vi "Find Names of PNP Devices.vi"(4 "Error In":errorcluster, 7 "Identifiers (regular expressions. Use blank to ignore)":T3={"Service"="FTSER2K", "Manufacturer"="FTDI", "Device"="FTDIBUS", "Vendor ID"="VID_0403", "Product ID"="PID_6001", "S/N"="FTXOVPUUA", "Instance"="0000"}) -> (0 "Error Out":errorcluster, 1 "Matching Items":T1(array[cluster]), 3 "Names":T2(array[cluster]))   [LabVIEW 2016]
doc: "Returns names, captions, & descriptions of PNP devices whose properties match the fields in the 'Identifiers' cluster\nFields are regular expressions (use .* to match any)."
uses:
  System.Management
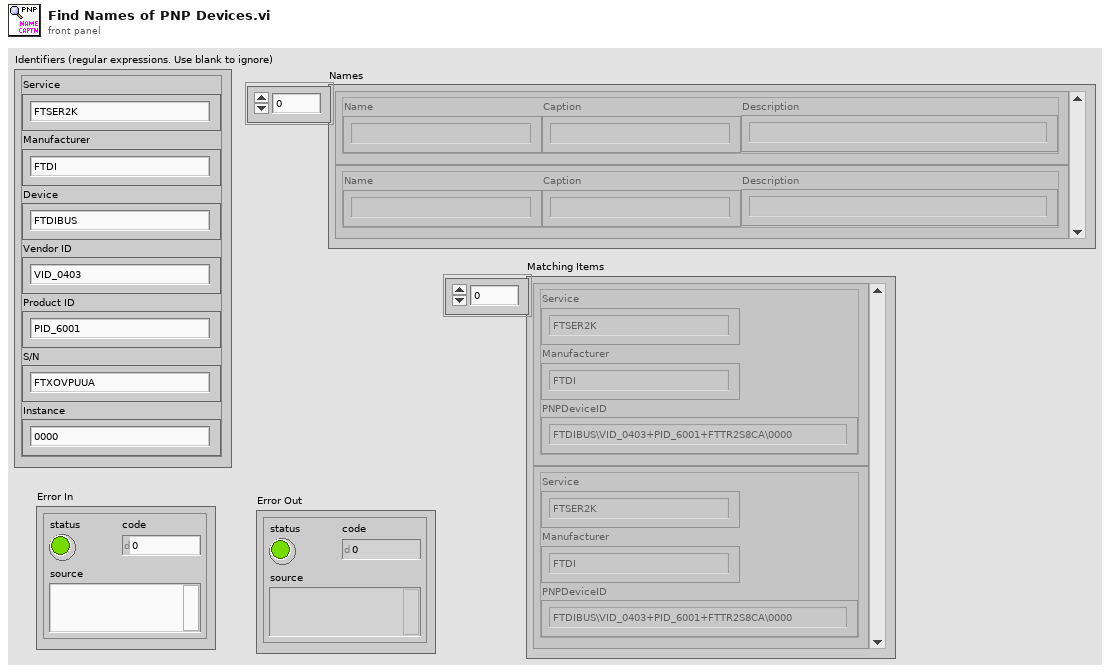
[diagram p1: front panel]
types:
  T1 = cluster{"Service":string, "Manufacturer":string, "PNPDeviceID":string}[]
  T2 = cluster{"Name":string, "Caption":string, "Description":string}[]
  T3 = cluster{"Service":string, "Manufacturer":string, "Device":string, "Vendor ID":string, "Product ID":string, "S/N":string, "Instance":string}
  T4 = cluster{"Property Values[0]":string, "Property Values[1]":string, "Property Values[2]":string}
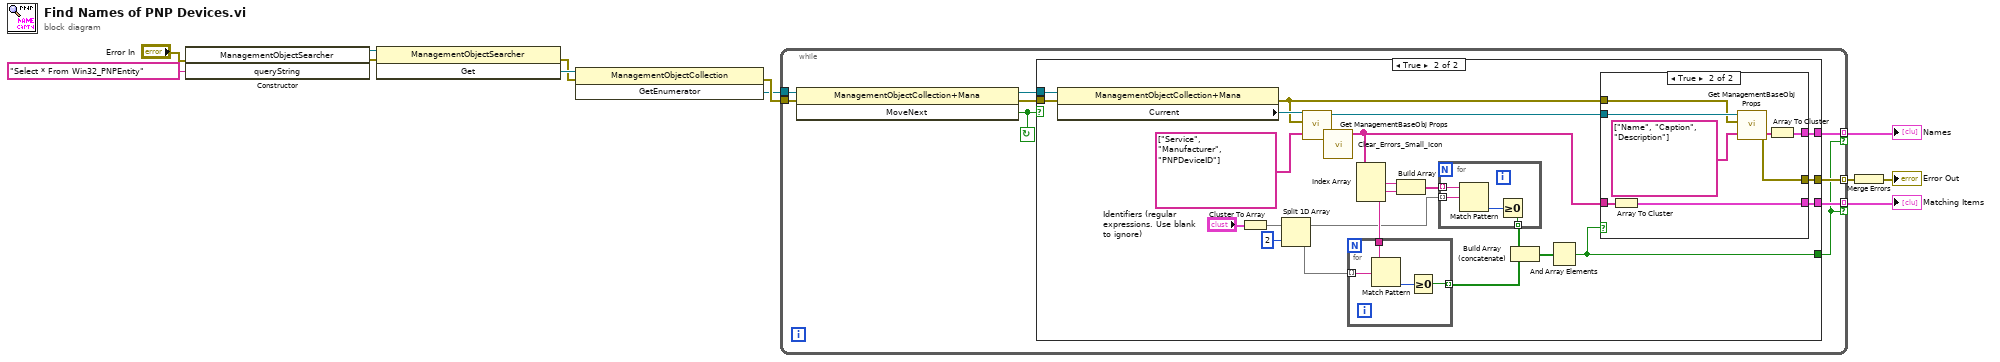
[diagram p0: block diagram]
diagram:
  n1 = constructor class="ManagementObjectSearcher"(error in="Error In", "queryString"="Select * From Win32_PNPEntity") -> (reference out=w8:refnum<k24>, error out=w7:errorcluster)  [unwired: 2 in, 2 out]
  n2 = invoke class="ManagementObjectSearcher" method="Get"(reference=w8, error in=w7) -> (error out=w9:errorcluster, "Get"=w10:refnum<k24>)  [unwired: 1 in, 1 out]
  n3 = invoke class="ManagementObjectCollection" method="GetEnumerator"(reference=w10, error in=w9) -> (error out=w12:errorcluster, "GetEnumerator"=w11:refnum<k24>)  [unwired: 1 in, 1 out]
  n4 = while {
    tunnel: [w21] -> w6 mode=indexing
    tunnel: w11 -> [w19]
    tunnel: w12 -> [w20]
    tunnel: [w15] -> w1 mode=indexing if=w13
    tunnel: [w14] -> w2 mode=indexing if=w13
    stop <- w16 continue-if-true
    n5 = invoke class="ManagementObjectCollection+Mana" method="MoveNext"(reference=w19, error in=w20) -> (reference out=w18:refnum<k24>, error out=w17:errorcluster, "MoveNext"=w16:bool)  [unwired: 1 in]
    n6 = case shown="True" w16 {
      tunnel: [w22 w28] -> w21
      tunnel: w18 -> [_ w46]
      tunnel: w17 -> [w22 w45]
      tunnel: [_ w29] -> w15
      tunnel: [_ w23] -> w13
      tunnel: [_ w39] -> w14
      frame False {
      }
      frame True {
        n7 = property class="ManagementObjectCollection+Mana"(reference=w46, error in=w45) -> (error out=w30:errorcluster, "Current"=w44:refnum<k24>)  [unwired: 1 out]
        n8 = Cluster To Array(cluster="Identifiers (regular expressions. Use blank to ignore)") -> (array=w38:string[])
        n9 = Split 1D Array(array=w38, index=2) -> (first subarray=w26:string[], second subarray=w24:string[])
        n10 = call "Get ManagementBaseObj Props.vi"(".NET Refnum in"=w44, "error in"=w30, "Property Names"=string[] ["Service", "Manufacturer", "PNPDeviceID"]) -> ("dup .NET Refnum"=w31:refnum<k24>, "error out"=w32:errorcluster, "Property Values"=w36:string[])  [unwired: 1 in]
        n11 = call "Clear_Errors_Small_Icon.vi"("error in (no error)"=w32) -> ()  [unwired: 6 in, 1 out]
        n12 = Index Array(array=w36) -> (element #1=w41:string, element #2=w40:string, element #3=w35:string)  [unwired: 3 in]
        n13 = for {
          tunnel: w35 -> [w59]
          tunnel: [w58] -> w34 mode=indexing
          tunnel: w24 -> [w56] mode=indexing
          n14 = Match Pattern(string=w59, regular expression=w56) -> (offset past match=w57:i32)  [unwired: 1 in, 3 out]
          n15 = Greater Or Equal To 0?(x=w57) -> (x >= 0?=w58:bool)
        }
        n16 = Build Array(w41, w40) -> (w27:string[])
        n17 = for {
          tunnel: [w63] -> w25 mode=indexing
          tunnel: w27 -> [w61] mode=indexing
          tunnel: w26 -> [w60] mode=indexing
          n18 = Match Pattern(string=w61, regular expression=w60) -> (offset past match=w62:i32)  [unwired: 1 in, 3 out]
          n19 = Greater Or Equal To 0?(x=w62) -> (x >= 0?=w63:bool)
        }
        n20 = Build Array (concatenate)(w25, w34) -> (w33:bool[])
        n21 = And Array Elements(Boolean array=w33) -> (logical AND=w23:bool)
        n22 = case shown="True" w23 {
          tunnel: [_ w55] -> w39
          tunnel: w36 -> [_ w54]
          tunnel: w31 -> [_ w53]
          tunnel: w30 -> [w47 w52]
          tunnel: [_ w48] -> w29
          tunnel: [w47 w51] -> w28
          frame False {
          }
          frame True {
            n23 = Array To Cluster(array=w54) -> (cluster=w55:T4)
            n24 = call "Get ManagementBaseObj Props.vi"(".NET Refnum in"=w53, "error in"=w52, "Property Names"=string[] ["Name", "Caption", "Description"]) -> ("error out"=w51:errorcluster, "Property Values"=w49:string[])  [unwired: 1 in, 1 out]
            n25 = Array To Cluster(array=w49) -> (cluster=w48:T4)
          }
        }
      }
    }
  }
  "Names" <- w1
  "Matching Items" <- w2
  n26 = Merge Errors(w6) -> (→"Error Out":errorcluster)
